vi "readBaseRecommendedSettings.vi"(8 "error in (no error)":errorcluster, 11 "Boot in":refnum<class "Boot.lvclass">) -> (0 "error out":errorcluster, 2 "RecommendedSettings":T1, 3 "Boot out":refnum<class "Boot.lvclass">)   [LabVIEW 2016, in "Boot.lvclass"]
uses:
  Boot.lvclass
  DataTypes/Settings/Base/RecommendedSettings.ctl
  Boot.lvclass/Boot.ctl
  Settings/Settings/Setting.lvclass
  DataTypes/Settings/M1M3SupportSettings.lvlib
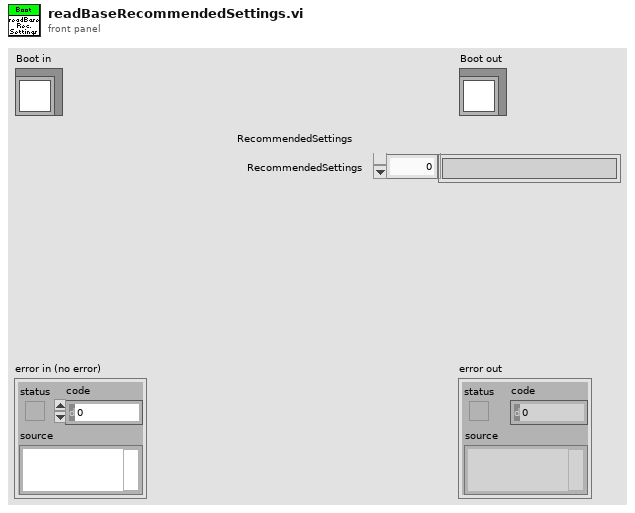
[diagram p1: front panel]
types:
  T1 = typedef "M1M3SupportSettings.lvlib/RecommendedSettings.ctl" = cluster{"RecommendedSettings":string[]}
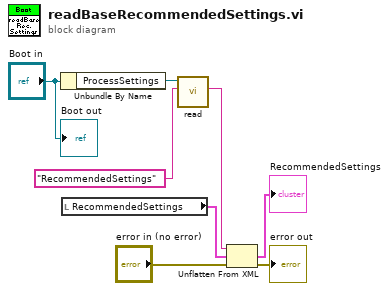
[diagram p0: block diagram]
diagram:
  n1 = Unbundle By Name("Boot in") -> ("ProcessSettings"=w8:refnum<class "Setting.lvclass">)
  n2 = local read "RecommendedSettings"() -> (w5:T1)
  n3 = call-dynamic "read.vi"("Name"="RecommendedSettings", "BaseSetting in"=w8) -> ("XML"=w7:string)  [unwired: 6 in, 3 out]
  n4 = Unflatten From XML(xml string=w7, type=w5, error in (no error)="error in (no error)") -> (value=→"RecommendedSettings":T1, error out=→"error out":errorcluster)
  "Boot out" <- "Boot in"
